vi "Stop.vi"(8 "error in (no error)":errorcluster, 9 "timeout in ms (-1)":i32=-1, 11 "Process In":refnum<class "Process.lvclass">) -> (0 "error out":errorcluster, 1 "timed out?":bool, 3 "Process Out":refnum<class "Process.lvclass">)   [LabVIEW 2020, in "Process.lvclass"]
doc: "Sends a stop message to the process, which must perform a safe shut down. This VI waits for the process to call the Finish method or times out if the configured time out expires. If the method does not time out, the process returned by this VI contains the full state of the process when it was stopped."
uses:
  Process.lvclass
  Process.lvclass/Process.ctl
  Public/Lifecycle/Lifecycle State.ctl
  Private/SubVIs/Handle Debug Data.vi
  Logging/Log Debug.vi
  <vilib>/AdvancedString/1D String Array to Delimited String.vi
  <vilib>/Utility/High Resolution Relative Seconds.vi
  <vilib>/Utility/error.llb/Error Cluster From Error Code.vi
  Public/Read Name.vi
  <vilib>/ErrorRing/Error Ring.xnode
  Callback/Callback.lvclass
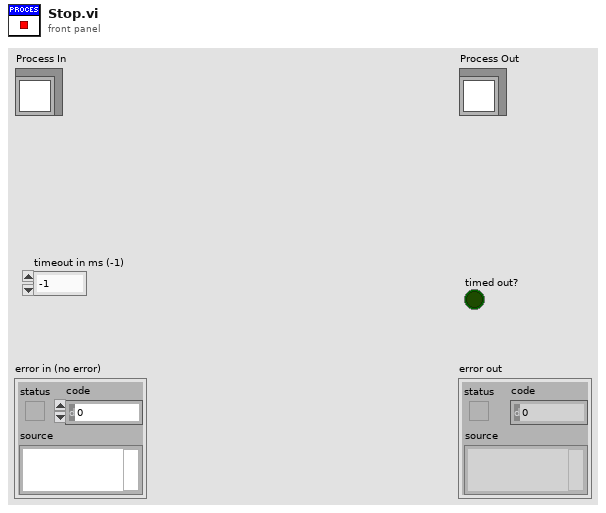
[diagram p1: front panel]
types:
  T1 = typedef "Process.lvclass/API Mode.ctl" = enum16{"Send Message", "Handle Message"}
  T2 = typedef "Process.lvclass/Lifecycle State.ctl" = enum16{"Uninitialized", "Initialized", "Started", "Running", "Stopped", "Finished"}
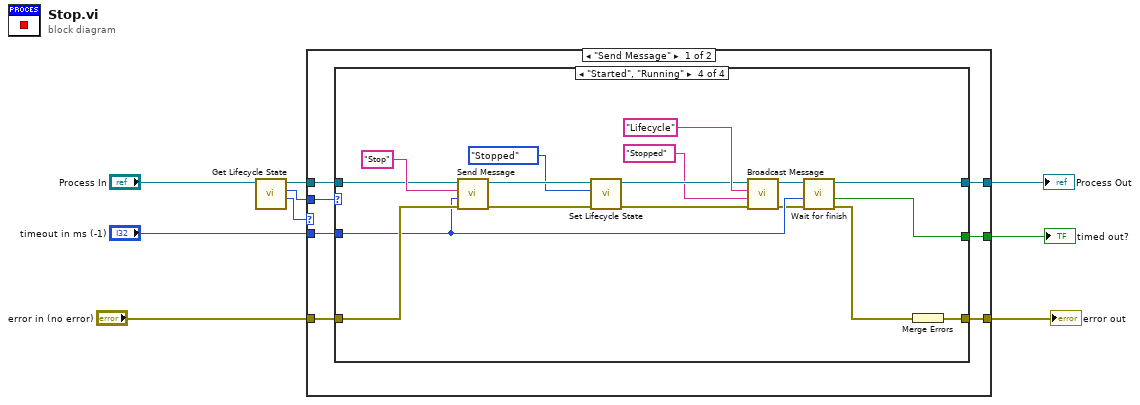
[diagram p0: block diagram]
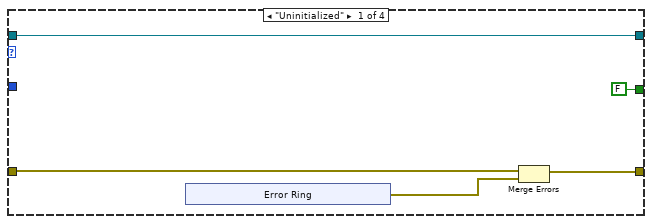
[diagram p2: hidden frame]
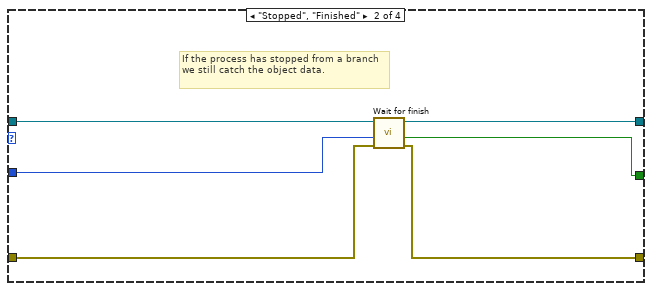
[diagram p3: hidden frame]
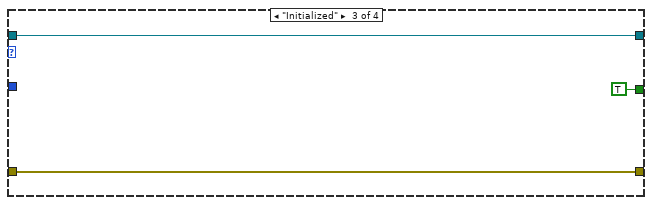
[diagram p4: hidden frame]
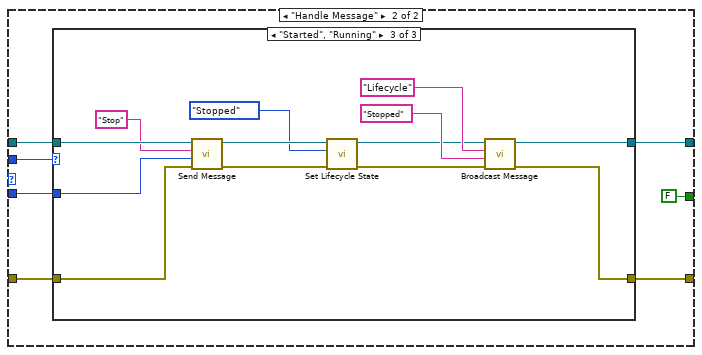
[diagram p5: hidden frame]
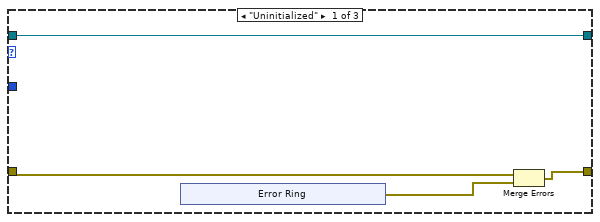
[diagram p6: hidden frame]
diagram:
  n1 = call "Get Lifecycle State.vi"("Process In"="Process In") -> ("API Mode"=w1:T1, "Lifecycle State"=w2:T2, "Process Out"=w3:refnum<class "Process.lvclass">)  [unwired: 7 in, 1 out]
  n2 = case shown="\"Send Message\"" w1 {
    tunnel: "timeout in ms (-1)" -> [w16 w54]
    tunnel: [w15 FALSE ("timed out?")] -> w7
    tunnel: [w14 w56] -> w6
    tunnel: [w13 w57] -> w5
    tunnel: w3 -> [w12 w52]
    tunnel: "error in (no error)" -> [w11 w58]
    tunnel: w2 -> [w10 w53]
    frame "Send Message" {
      n3 = case shown="\"Started\", \"Running\"" w10 {
        tunnel: w16 -> [_ w29 _ w42]
        tunnel: [FALSE ("timed out?") w26 TRUE ("timed out?") w51] -> w15
        tunnel: [w18 w28 w33 w47] -> w14
        tunnel: [w21 w31 w34 w46] -> w13
        tunnel: w12 -> [w21 w30 w34 w45]
        tunnel: w11 -> [w17 w27 w33 w44]
        frame "Uninitialized" {
          n4 = xnode "Error Ring"() -> ("error out"=w19:errorcluster)
          n5 = Merge Errors(w17, w19) -> (w18:errorcluster)
        }
        frame "Stopped", "Finished" {
          # "If the process has stopped from a branch we still catch the object data."
          n6 = call "Wait for finish.vi"("error in (no error)"=w27, "timeout in ms (-1)"=w29, "Process In"=w30) -> ("error out"=w28:errorcluster, "timed out?"=w26:bool, "Process Out"=w31:refnum<class "Process.lvclass">)  [unwired: 6 in]
        }
        frame "Initialized" {
        }
        frame "Started", "Running" {
          n7 = call "Send Message.vi"("error in (no error)"=w44, "Message Data"=w42, "Message"="Stop", "Process In"=w45) -> ("error out"=w43:errorcluster, "Process Out"=w48:refnum<class "Process.lvclass">)  [unwired: 6 in]
          n8 = call "Set Lifecycle State.vi"("error in (no error)"=w43, "Lifecycle State"=Lifecycle_State."Stopped", "Process In"=w48) -> ("error out"=w39:errorcluster, "Process Out"=w36:refnum<class "Process.lvclass">)  [unwired: 7 in]
          n9 = call-dynamic "Broadcast Message.vi"("error in (no error)"=w39, "Message Data"="Stopped" ("Message"), "Message"="Lifecycle", "Process In"=w36) -> ("error out"=w38:errorcluster, "Process Out"=w37:refnum<class "Process.lvclass">)  [unwired: 6 in]
          n10 = call "Wait for finish.vi"("error in (no error)"=w38, "timeout in ms (-1)"=w42, "Process In"=w37) -> ("error out"=w50:errorcluster, "timed out?"=w51:bool, "Process Out"=w46:refnum<class "Process.lvclass">)  [unwired: 6 in]
          n11 = Merge Errors(w50) -> (w47:errorcluster)
        }
      }
    }
    frame "Handle Message" {
      n12 = case shown="\"Started\", \"Running\"" w53 {
        tunnel: w52 -> [w59 w67 w81]
        tunnel: w58 -> [w61 w68 w80]
        tunnel: [w59 w67 w69] -> w57
        tunnel: [w60 w68 w71] -> w56
        tunnel: w54 -> [_ _ w75]
        frame "Uninitialized" {
          n13 = xnode "Error Ring"() -> ("error out"=w62:errorcluster)
          n14 = Merge Errors(w61, w62) -> (w60:errorcluster)
        }
        frame "Initialized", "Stopped", "Finished" {
        }
        frame "Started", "Running" {
          n15 = call "Send Message.vi"("error in (no error)"=w80, "Message Data"=w75, "Message"="Stop", "Process In"=w81) -> ("error out"=w78:errorcluster, "Process Out"=w79:refnum<class "Process.lvclass">)  [unwired: 6 in]
          n16 = call "Set Lifecycle State.vi"("error in (no error)"=w78, "Lifecycle State"=Lifecycle_State."Stopped", "Process In"=w79) -> ("error out"=w72:errorcluster, "Process Out"=w70:refnum<class "Process.lvclass">)  [unwired: 7 in]
          n17 = call-dynamic "Broadcast Message.vi"("error in (no error)"=w72, "Message Data"="Stopped" ("Message"), "Message"="Lifecycle", "Process In"=w70) -> ("error out"=w71:errorcluster, "Process Out"=w69:refnum<class "Process.lvclass">)  [unwired: 6 in]
        }
      }
    }
  }
  "error out" <- w6
  "Process Out" <- w5
  "timed out?" <- w7
